vi "Read_ProcessID.vi"(8 "error in (no error)":errorcluster, 11 "Process in":refnum<class "Process.lvclass">) -> (0 "error out":errorcluster, 2 "Process":T1, 3 "Process out":refnum<class "Process.lvclass">)   [LabVIEW 2013, in "Process.lvclass"]
uses:
  Process.lvclass
  EnumProcess.ctl
  Process.lvclass/Process.ctl
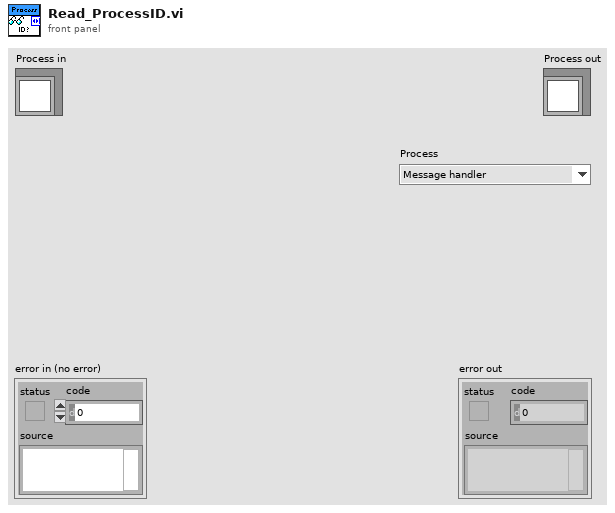
[diagram p1: front panel]
types:
  T1 = typedef "Process.lvclass/EnumProcess.ctl" = enum16{"Message handler", "Template"}
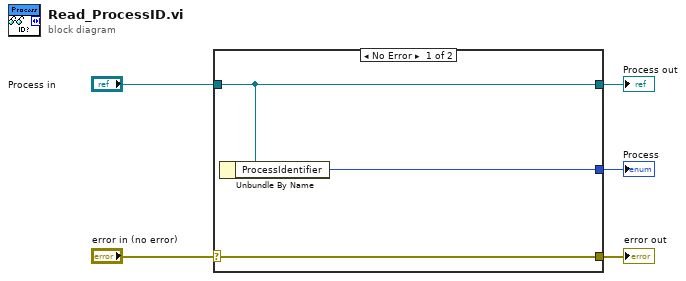
[diagram p0: block diagram]
diagram:
  n1 = case shown="No Error" "error in (no error)" {
    selector: "error in (no error)" -> [w8 w9]
    tunnel: [w8 w9] -> w4
    tunnel: [w7 w10] -> w2
    tunnel: "Process in" -> [w7 w10]
    tunnel: [w6 _] -> w1
    frame No Error {
      n2 = Unbundle By Name(w7) -> ("ProcessIdentifier"=w6:T1)
    }
    frame Error {
    }
  }
  "error out" <- w4
  "Process out" <- w2
  "Process" <- w1
